vi "Example Launcher.vi"   [LabVIEW 2016]
uses:
  Example Source/Example Source/Example Source.lvclass
  C:/Projects/Shared Libraries/Event Actors/Examples/Timed Loop Controller/Timed Loop Controller/Timed Loop Controller.lvclass
  C:/Program Files (x86)/National Instruments/LabVIEW 2016/vi.lib/ActorFramework/Actor/Actor.lvclass
  Timed Loop Controller/Timed Loop Controller/Timed Loop Controller.lvclass
  <vilib>/ActorFramework/Actor/Actor.lvclass
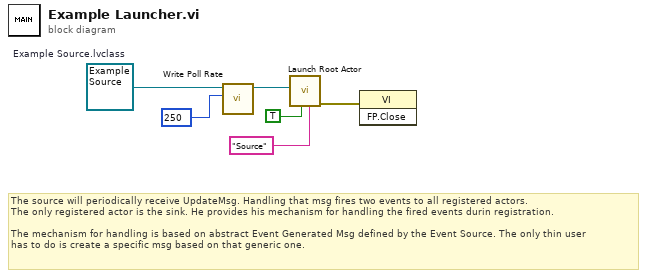
[diagram p0: block diagram]
diagram:
  w6 = refnum<class "Example Source.lvclass"> refnum  # Example Source.lvclass
  # "The source will periodically receive UpdateMsg. Handling that msg fires two events to all registered actors.\nThe only registered actor is the sink. He provides his mechanism for handling the fired events durin registration.\n\nThe mechanism for handling is based on abstract Event Generated Msg defined by the Event Source. The only thin user\nhas to do is create a specific msg based on that generic one."
  n1 = call "Write Poll Rate.vi"("Poll Rate"=u32 250, "Timed Loop Controller in"=w6) -> ("Timed Loop Controller out"=w5:refnum<class "Example Source.lvclass">)  [unwired: 8 in, 1 out]
  n2 = call <vilib>:"Launch Root Actor.vi"("Debug Alias"="Source", "Open Actor Core front panel? (F)"=TRUE, "Actor"=w5) -> ("error out"=w3:errorcluster)  [unwired: 7 in, 1 out]
  n3 = invoke class="VI" method="FP.Close"(error in=w3) -> ()  [unwired: 2 in, 3 out]
